vi "Set Port Parameters.vi"(8 "error in (no error)":errorcluster, 10 "Port Parameters":T1={"Bytes to Read"=1000, "Line Separator"="\n", "Port Timeout (ms)"=5000, "Read Mode"=enum."normal", "Write Mode"=enum."normal", "Remote Port"=23}, 11 "niDTS Comm Telnet in":refnum<class "niDTS Comm Telnet.lvclass">) -> (0 "error out":errorcluster, 3 "niDTS Comm Telnet out":refnum<class "niDTS Comm Telnet.lvclass">)   [LabVIEW 2015, in "niDTS CommLib.lvlib" / "niDTS Comm Telnet.lvclass"]
uses:
  niDTS Comm Telnet.lvclass
  Includes/niDTS Comm INC Telnet Port Parameters.ctl
  niDTS Comm Telnet.lvclass/niDTS Comm Telnet.ctl
  niDTS CommLib.lvlib
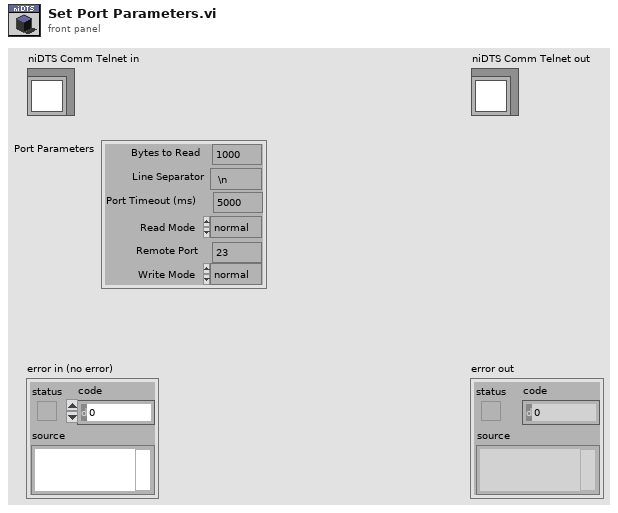
[diagram p1: front panel]
types:
  T1 = typedef "niDTS CommLib.lvlib/niDTS Comm INC Telnet Port Parameters.ctl" = cluster{"Bytes to Read":i32, "Line Separator":string, "Port Timeout (ms)":i32, "Read Mode":enum16{"normal", "line", "buffered"}, "Write Mode":enum16{"normal", "line", "buffered"}, "Remote Port":u16}
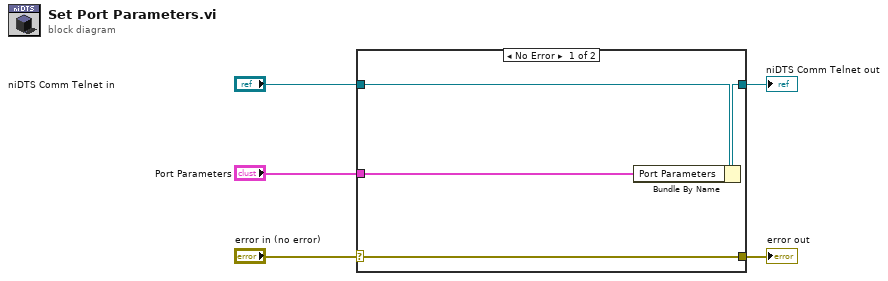
[diagram p0: block diagram]
diagram:
  n1 = case shown="No Error" "error in (no error)" {
    selector: "error in (no error)" -> [w9 w10]
    tunnel: [w9 w10] -> w4
    tunnel: [w7 w11] -> w2
    tunnel: "niDTS Comm Telnet in" -> [w8 w11]
    tunnel: "Port Parameters" -> [w6 _]
    frame No Error {
      n2 = Bundle By Name(cluster=w8, "Port Parameters"=w6) -> (w7:refnum<class "niDTS Comm Telnet.lvclass">)
    }
    frame Error {
    }
  }
  "error out" <- w4
  "niDTS Comm Telnet out" <- w2
